vi "getAllStatusBits.vi"(8 "error in (no error)":errorcluster, 10 "Axis Letter":string, 11 "Controller.LV in":refnum<class "Controller.LV.lvclass">) -> (0 "error out":errorcluster, 2 "STAT":string, 3 "Controller.LV out":refnum<class "Controller.LV.lvclass">)   [LabVIEW 2019, in "Controller.LV.lvclass"]
uses:
  Controller.LV.lvclass
  drivers/Class/Axis/Axis.lvclass
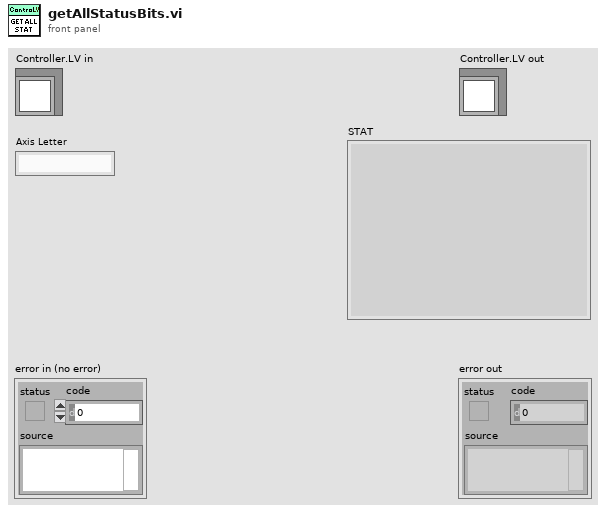
[diagram p1: front panel]
types:
  T1 = cluster{"SRNO":dbl, "SOFT":dbl, "STAT":dbl, "FREQ":dbl, "OFRQ":dbl, "CURR":dbl, "SYNC":dbl, "Encoder Position [enc. units]":dbl, "Desired Position [enc. units]":dbl, "TIME":dbl}
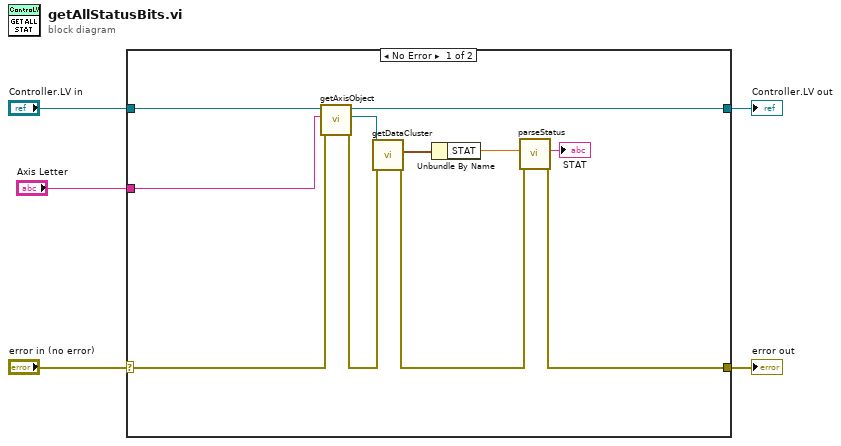
[diagram p0: block diagram]
diagram:
  n1 = case shown="No Error" "error in (no error)" {
    selector: "error in (no error)" -> [w14 w18]
    tunnel: [w13 w18] -> w4
    tunnel: [w16 w17] -> w2
    tunnel: "Controller.LV in" -> [w15 w17]
    tunnel: "Axis Letter" -> [w7 _]
    frame No Error {
      n2 = call-dynamic "getAxisObject.vi"("error in (no error)"=w14, "Axis Letter"=w7, "Controller in"=w15) -> ("error out"=w11:errorcluster, "Axis Object"=w12:refnum<class "Axis.lvclass">, "Controller out"=w16:refnum<class "Controller.LV.lvclass">)  [unwired: 6 in]
      n3 = call-dynamic "getDataCluster.vi"("error in (no error)"=w11, "Axis in"=w12) -> ("error out"=w9:errorcluster, "Information"=w10:T1)  [unwired: 7 in, 1 out]
      n4 = Unbundle By Name(w10) -> ("STAT"=w8:dbl)
      n5 = call "parseStatus.vi"("error in"=w9, "STAT word"=w8) -> ("error out"=w13:errorcluster, "Status"=→"STAT":string)  [unwired: 8 in]
    }
    frame Error {
    }
  }
  "error out" <- w4
  "Controller.LV out" <- w2
